vi "Tree Get Selected Indices.vi"(8 "error in (no error)":errorcluster, 11 "Tree Ref":refnum<vi>) -> (0 "error out":errorcluster, 1 "Tree.Values":string[](array[string]), 2 "Selected Indices":i32[](array[numeric]), 3 "tree ref":refnum<vi>, 4 "Tree.All Tags":string[](array[string]))   [LabVIEW 2020, in "BetterDragAndDrop.lvlib" / "BetterTreeHandle.lvclass"]
uses:
  Classes/BetterTreeHandle/BetterTreeHandle.lvclass
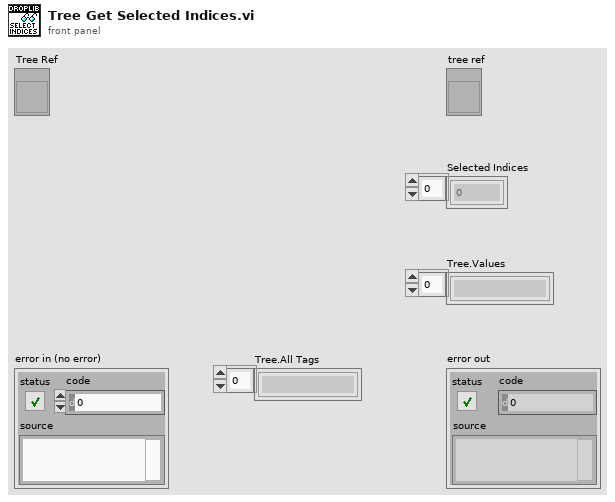
[diagram p1: front panel]
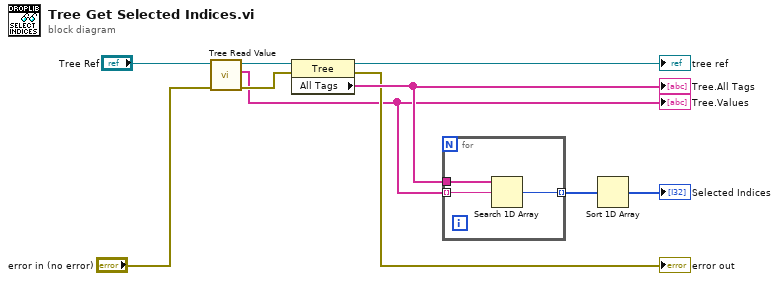
[diagram p0: block diagram]
diagram:
  n1 = call "Tree Read Value.vi"("error in (no error)"="error in (no error)", "Tree Ref (generic)"="Tree Ref") -> ("error out"=w2:errorcluster, "Value"=w1:string[], "Tree Ref (generic)"=w4:refnum<vi>)  [unwired: 7 in]
  "Tree.Values" <- w1
  n2 = property class="Tree"(reference=w4, error in=w2) -> (reference out=→"tree ref":refnum<vi>, error out=→"error out":errorcluster, "All Tags"=w9:string[])
  "Tree.All Tags" <- w9
  n3 = for {
    tunnel: w1 -> [w13] mode=indexing
    tunnel: w9 -> [w12]
    tunnel: [w11] -> w10 mode=indexing
    n4 = Search 1D Array(1D array=w12, element=w13) -> (index of element=w11:i32)  [unwired: 1 in]
  }
  n5 = Sort 1D Array(array=w10) -> (sorted array=→"Selected Indices":i32[])
